vi "Actor Core.vi"(8 "error in":errorcluster, 11 "Root Tester in":refnum<class "Root Tester.lvclass">) -> (0 "error out":errorcluster, 3 "Actor out":refnum<class "Actor.lvclass">)   [LabVIEW 2024, in "Root Tester.lvlib" / "Root Tester.lvclass"]
doc: "<p>(<strong>Filename</strong>: <span class=\"dnl\">Actor Framework.lvlib:Actor.lvclass:Actor Core.vi</span>)</p>\n<p>Receives messages to the actor, reacts to them, and initiates any error handling that may shut the actor down.</p>\n<p>Descendant classes may override this VI to append parallel tasks for the actor to complete while it handles messages. Overrides use the <a href=\"nihelplauncher://docs/csh?context=lvcore_glang_udclass\">Call Parent Class Method</a> node.</p>"
uses:
  Root Tester.lvclass
  C:/Program Files (x86)/National Instruments/LabVIEW 2024/vi.lib/ActorFramework/Actor/Actor.lvclass
  <vilib>/ActorFramework/Actor/Actor.lvclass
  <vilib>/ActorFramework/Actor/Actor.lvclass/Actor.ctl
  <vilib>/ActorFramework/Message Enqueuer/Message Enqueuer.lvclass/Message Enqueuer.ctl
  Root Tester.lvclass/Root Tester.ctl
  <vilib>/ActorFramework/Message Enqueuer/Init from Existing Queue.vi
  <vilib>/ActorFramework/Message Enqueuer/Enqueue.vi
  <vilib>/ActorFramework/Stop Msg/Stop Msg.lvclass
  C:/Program Files (x86)/National Instruments/LabVIEW 2024/vi.lib/ActorFramework/Message/Message.lvclass
  <vilib>/measure/macond.llb/IIR Filter for N Chan.vi
  <vilib>/ActorFramework/Message Priority Queue/Priority Enqueue.vi
  <vilib>/ActorFramework/Message Enqueuer/Message Enqueuer.lvclass
  <vilib>/measure/NI_MAPro.lvlib
  DAQmx Actor/Digital Writer Messages/Digital Write Multiple Msg/Digital Write Multiple Msg.lvclass
  C:/Users/uspoaotto/OneDrive - Oregon Tool/Desktop/working copies/DAQmxActor/src/Root Tester/Root Tester/Root Tester.lvclass
  C:/Users/uspoaotto/OneDrive - Oregon Tool/Desktop/working copies/DAQmxActor/src/DAQmx Actor Interface/Analog Input Waveform Data/Analog Input Waveform Data.lvclass
  C:/Users/uspoaotto/OneDrive - Oregon Tool/Desktop/working copies/DAQmxActor/src/DAQmx Actor Interface/Digital Input Data/Digital Input Data.lvclass
panel:
  in  "Digital Outputs":enum32{"on", "off"}[][](array[radio])=[[enum."off", enum."off", enum."off", enum."off"], [enum."off", enum."off", enum."off", enum."off"]]
  out "Analog Inputs":dbl[](array[numeric])
  out "Digital Inputs":bool[](array[boolean])
  out "Digital Inputs":i16[][](graph)
  out "ESTOP":bool
  out "Analog Inputs":waveform(dbl)[](graph)
  in  "Stop":bool
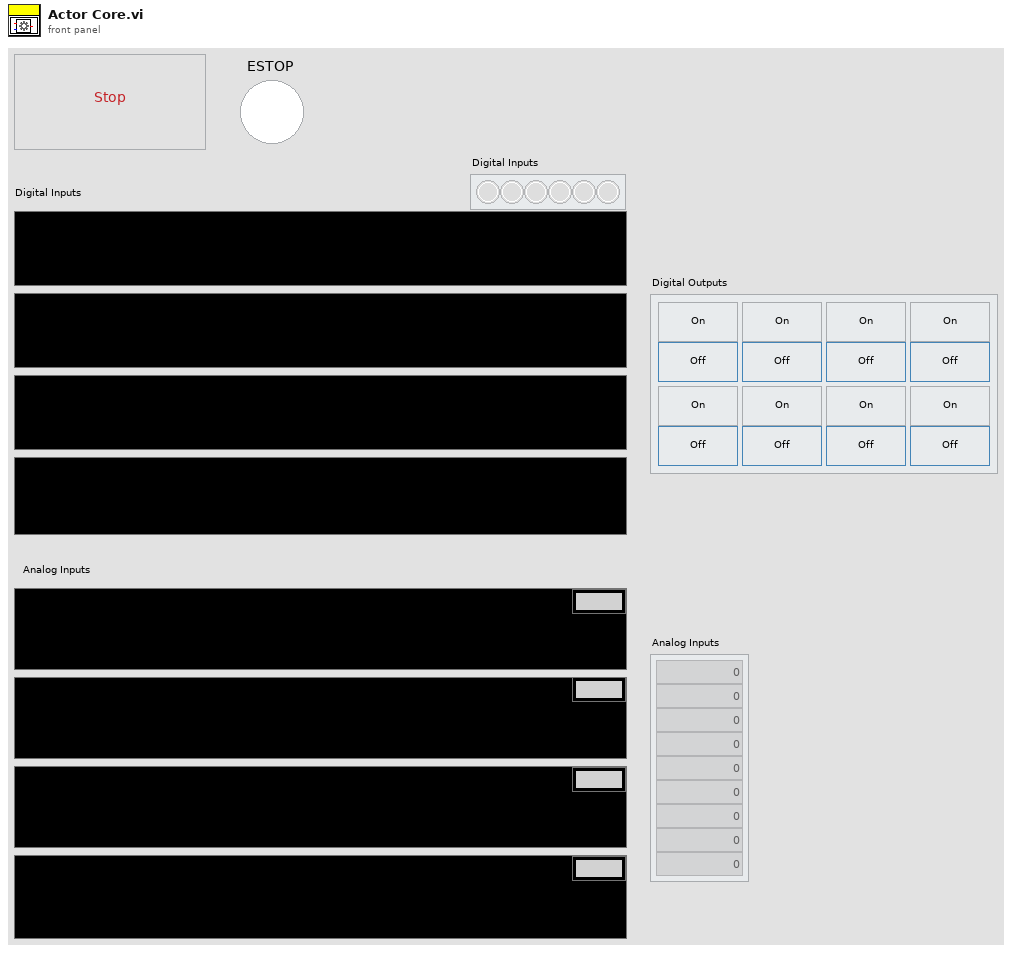
[diagram p1: front panel]
types:
  T1 = cluster{"Topology":enum16{"Off", "Butterworth", "Chebyshev", "Inverse Chebyshev", "Elliptic", "Bessel"}, "Type":enum16{"Lowpass", "Highpass", "Bandpass", "Bandstop"}, "Order":i32, "Lower Fc":dbl, "Upper Fc":dbl, "PB Ripple":dbl, "SB Attenuation":dbl}
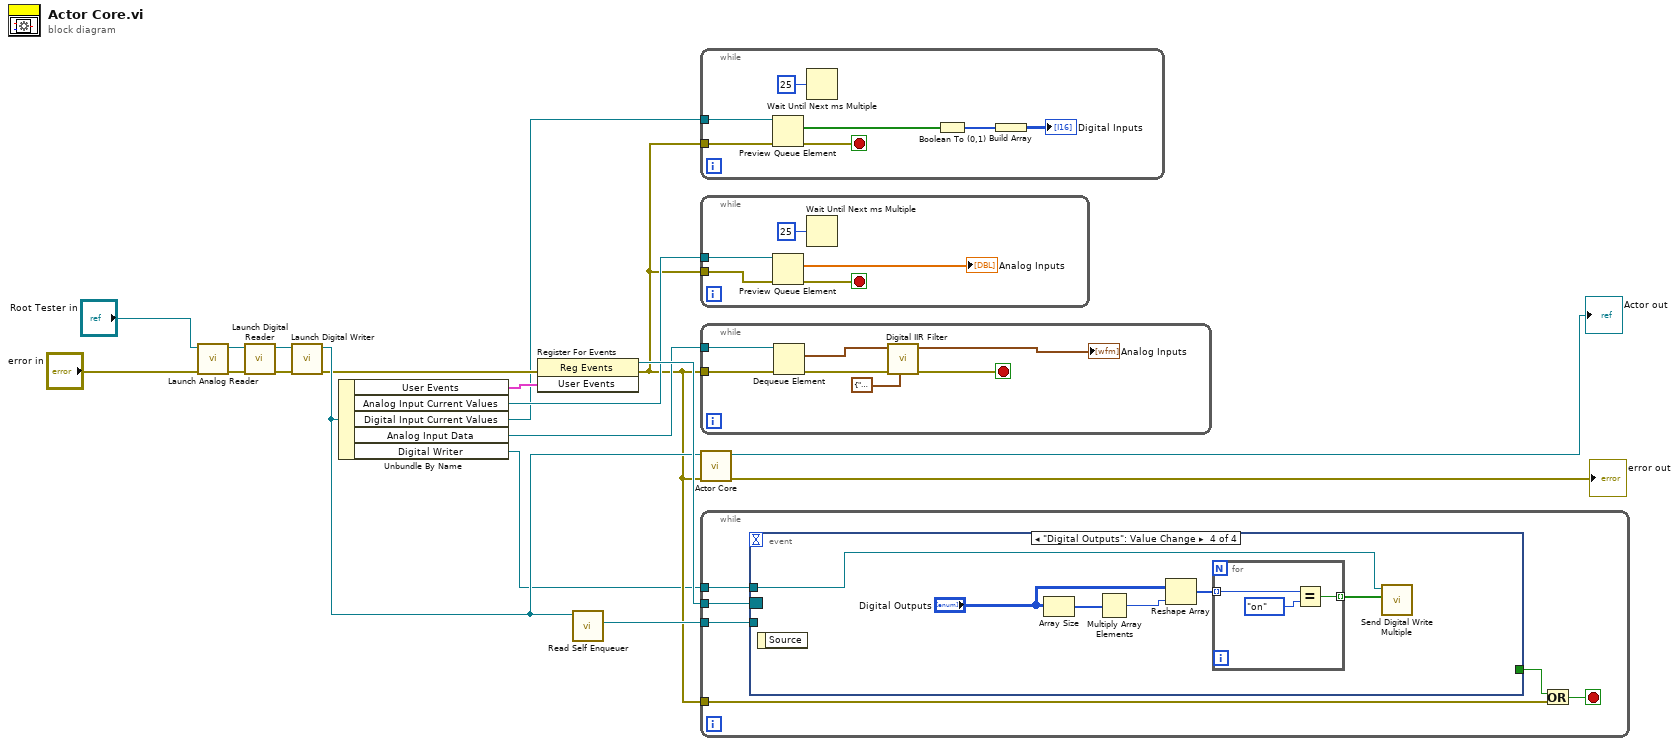
[diagram p0: block diagram]
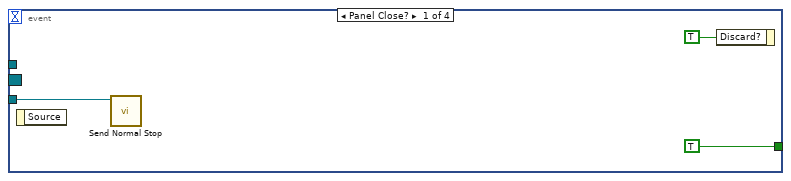
[diagram p2: hidden frame]
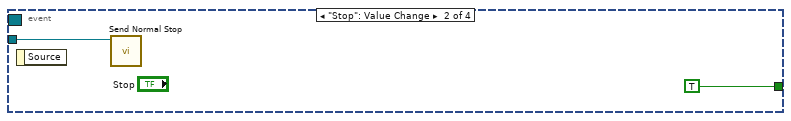
[diagram p3: hidden frame]
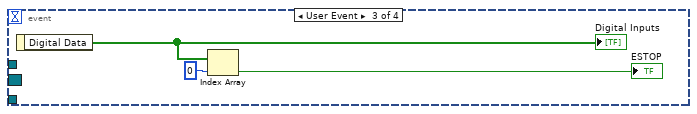
[diagram p4: hidden frame]
diagram:
  n1 = call-dynamic "Launch Analog Reader.vi"("error in (no error)"="error in", "Root Tester in"="Root Tester in") -> ("error out"=w10:errorcluster, "Root Tester out"=w12:refnum<class "Root Tester.lvclass">)  [unwired: 8 in]
  n2 = call-dynamic "Launch Digital Reader.vi"("error in (no error)"=w10, "Root Tester in"=w12) -> ("error out"=w7:errorcluster, "Root Tester out"=w9:refnum<class "Root Tester.lvclass">)  [unwired: 8 in]
  n3 = call-dynamic "Launch Digital Writer.vi"("error in (no error)"=w7, "Root Tester in"=w9) -> ("error out"=w6:errorcluster, "Root Tester out"=w8:refnum<class "Root Tester.lvclass">)  [unwired: 8 in]
  n4 = Unbundle By Name(w8) -> ("User Events"=w15:cluster{"Digital Data":refnum<user-event>}, "Analog Input Current Values"=w5:refnum<queue>, "Digital Input Current Values"=w4:refnum<queue>, "Analog Input Data"=w3:refnum<queue>, "Digital Writer"=w1:refnum<class "Message Enqueuer.lvclass">)
  n5 = register-events(error in=w6, w15) -> (reference out=w14:refnum<event-registration>, error out=w2:errorcluster)  [unwired: 1 in]
  n6 = call <vilib>:"Read Self Enqueuer.vi"("Actor"=w8) -> ("Self Enqueuer"=w16:refnum<class "Message Enqueuer.lvclass">)  [unwired: 10 in]
  n7 = while {
    tunnel: w4 -> [w25]
    tunnel: w2 -> [w24]
    stop <- w23 stop-if-true
    n8 = Preview Queue Element(queue=w25, error in (no error)=w24) -> (element=w21:bool[], error out=w23:errorcluster)  [unwired: 1 in, 2 out]
    n9 = Wait Until Next ms Multiple(millisecond multiple=u32 25) -> ()  [unwired: 1 out]
    n10 = Boolean To (0,1)(Boolean=w21) -> (0, 1=w20:i16[])
    n11 = Build Array(w20) -> (→"Digital Inputs":i16[][])
  }
  n12 = while {
    tunnel: w5 -> [w30]
    tunnel: w2 -> [w29]
    stop <- w28 stop-if-true
    n13 = Preview Queue Element(queue=w30, error in (no error)=w29) -> (element=→"Analog Inputs":dbl[], error out=w28:errorcluster)  [unwired: 1 in, 2 out]
    n14 = Wait Until Next ms Multiple(millisecond multiple=u32 25) -> ()  [unwired: 1 out]
  }
  n15 = while {
    tunnel: w3 -> [w37]
    tunnel: w2 -> [w36]
    stop <- w31 stop-if-true
    n16 = Dequeue Element(queue=w37, error in (no error)=w36) -> (element=w33:waveform(dbl)[], error out=w32:errorcluster)  [unwired: 1 in, 2 out]
    n17 = call-poly <vilib>:"Digital IIR Filter.vi"("IIR filter specifications"=T1 {"Topology"=enum."Bessel", "Type"=enum."Lowpass", "Order"=5, "Lower Fc"=10.0, "Upper Fc"=10.0, "PB Ripple"=1.0, "SB Attenuation"=60.0}, "error in (no error)"=w32, "signal(s) in"=w33) -> ("error out"=w31:errorcluster, "signal(s) out"=→"Analog Inputs":waveform(dbl)[])  [unwired: 6 in, 1 out]
  }
  n18 = call-parent "Actor Core.vi"("error in"=w2, "Actor in"=w8) -> ("error out"=→"error out":errorcluster, "Actor out"=→"Actor out":refnum<class "Actor.lvclass">)  [unwired: 8 in]
  n19 = while {
    tunnel: w16 -> [w43]
    tunnel: w14 -> [w42]
    tunnel: w2 -> [w40]
    tunnel: w1 -> [w38]
    stop <- w39 stop-if-true
    n20 = event shown="[3] \"Digital Outputs\": Value Change" {
      selector: w42 -> [_ _ _ _]
      dyn-events: _ -> [_ _ _ _]
      timeout: _ -> [_ _ _ _]
      tunnel: w43 -> [w46 w47 _ _]
      tunnel: [TRUE TRUE _ _] -> w41
      tunnel: w38 -> [_ _ _ w52]
      event Panel Close? {
        n21 = event-data() -> ()  [unwired: 1 in, 1 out]
        n22 = call <vilib>:"Send Normal Stop.vi"("Message Enqueuer"=w46) -> ()  [unwired: 10 in, 1 out]
        n23 = event-data("Discard?"=TRUE) -> ()  [unwired: 1 in, 1 out]
      }
      event "Stop": Value Change {
        n24 = event-data() -> ()  [unwired: 1 in, 1 out]
        n25 = call <vilib>:"Send Normal Stop.vi"("Message Enqueuer"=w47) -> ()  [unwired: 10 in, 1 out]
      }
      event User Event {
        n26 = event-data() -> ("Digital Data"=w49:bool[])  [unwired: 1 in]
        "Digital Inputs" <- w49
        n27 = Index Array(array=w49, index=0) -> (element=→"ESTOP":bool)
      }
      event "Digital Outputs": Value Change {
        n28 = event-data() -> ()  [unwired: 1 in, 1 out]
        n29 = Array Size(array="Digital Outputs") -> (size(s)=w57:i32[])
        n30 = Multiply Array Elements(1:w57) -> (0:w56:i32)
        n31 = Reshape Array("Digital Outputs", w56) -> (w54:enum32{"on", "off"}[])
        n32 = for {
          tunnel: w54 -> [w60] mode=indexing
          tunnel: [w58] -> w53 mode=indexing
          n33 = Equal?(x=w60, y=enum32{"on", "off"}."on") -> (x = y?=w58:bool)
        }
        n34 = call "Send Digital Write Multiple.vi"("Digital Data"=w53, "Message Enqueuer"=w52) -> ()  [unwired: 8 in, 2 out]
      }
    }
    n35 = Or(x=w41, y=w40) -> (x .or. y?=w39:bool)
  }
